vi "createSegment.vi"(4 "log":string, 5 "time":string, 6 "Parameter":string[][](array[string]), 7 "Comment":string, 8 "error in (no error)":errorcluster, 9 "SegName":string, 10 "test ref":refnum<k20>, 11 "DOM document":refnum<k20>) -> (0 "error out":errorcluster, 1 "seg ref":refnum<k20>, 2 "dup test ref":refnum<k20>, 3 "dup DOM document":refnum<k20>)   [LabVIEW 2013, in "XML.lvlib"]
uses:
  lib/XML.lvlib
  <vilib>/xml/Close Reference(Node).vi
  <resource>/objmgr/DOMUserDefRef.rc
  <vilib>/xml/NI_XML.lvlib
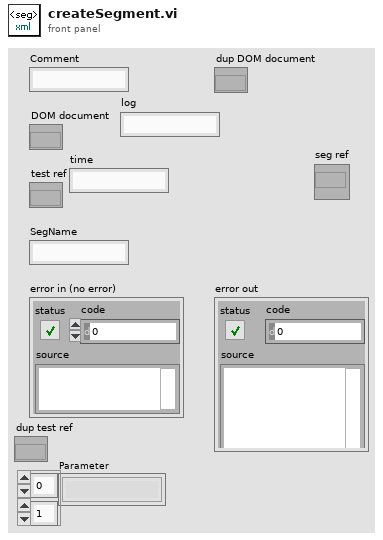
[diagram p1: front panel]
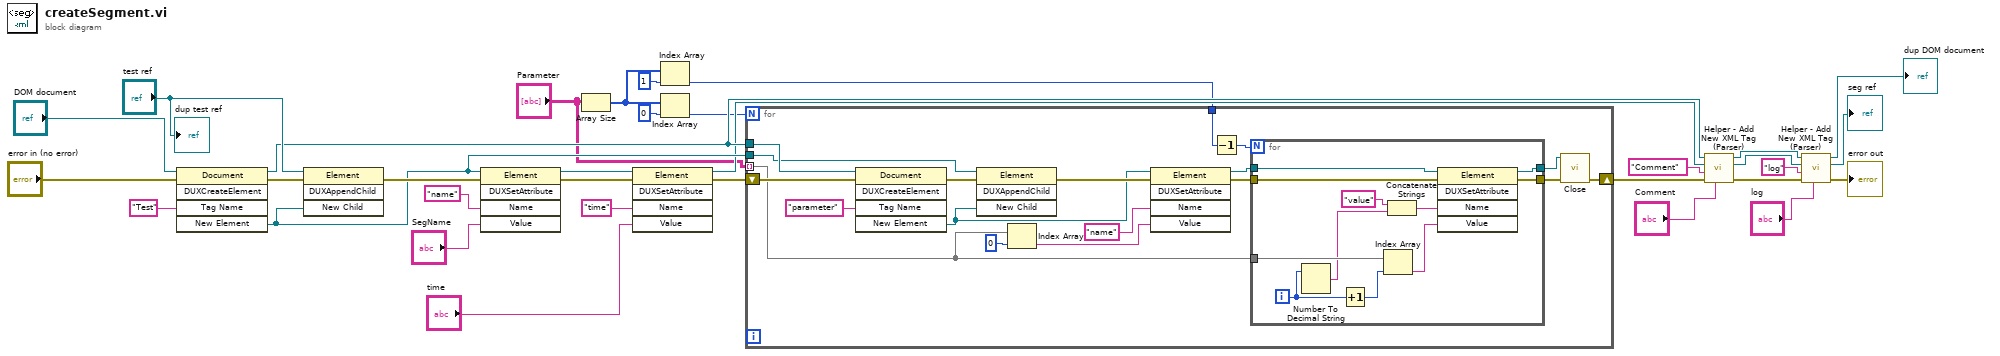
[diagram p0: block diagram]
diagram:
  n1 = invoke class="Document" method="DUXCreateElement"(reference="DOM document", error in="error in (no error)", "Tag Name"="Test") -> (reference out=w11:refnum<k20>, error out=w31:errorcluster, "New Element"=w8:refnum<k20>)  [unwired: 2 in, 2 out]
  n2 = invoke class="Element" method="DUXAppendChild"(reference="test ref", error in=w31, "New Child"=w8) -> (error out=w27:errorcluster)  [unwired: 1 in, 3 out]
  n3 = invoke class="Element" method="DUXSetAttribute"(reference=w8, error in=w27, "Name"="name" ("Tag Name"), "Value"="SegName") -> (reference out=w22:refnum<k20>, error out=w23:errorcluster)  [unwired: 1 in, 3 out]
  n4 = Array Size(array="Parameter") -> (size(s)=w2:i32[])
  n5 = invoke class="Element" method="DUXSetAttribute"(reference=w22, error in=w23, "Name"="time" ("Tag Name"), "Value"="time") -> (reference out=w7:refnum<k20>, error out=w10:errorcluster)  [unwired: 1 in, 3 out]
  n6 = Index Array(array=w2, index=1 ("Index")) -> (element=w1:i32)
  n7 = Index Array(array=w2, index=0 ("Index")) -> (element=w4:i32)
  n8 = for {
    N: w4 -> [_]
    tunnel: "Parameter" -> [w36] mode=indexing
    tunnel: w11 -> [w45]
    shift-right: [w37] -> w9
    shift-left: w10 -> [w44]
    tunnel: w8 -> [w43]
    tunnel: w1 -> [w34]
    n9 = invoke class="Document" method="DUXCreateElement"(reference=w45, error in=w44, "Tag Name"="parameter") -> (error out=w50:errorcluster, "New Element"=w42:refnum<k20>)  [unwired: 2 in, 3 out]
    n10 = invoke class="Element" method="DUXAppendChild"(reference=w43, error in=w50, "New Child"=w42) -> (error out=w46:errorcluster)  [unwired: 1 in, 3 out]
    n11 = Index Array(array=w36, index=0 ("Index")) -> (element=w40:string)
    n12 = invoke class="Element" method="DUXSetAttribute"(reference=w42, error in=w46, "Name"="name" ("Tag Name"), "Value"=w40) -> (reference out=w49:refnum<k20>, error out=w48:errorcluster)  [unwired: 1 in, 3 out]
    n13 = Decrement(x=w34) -> (x-1=w35:i32)
    n14 = for {
      N: w35 -> [_]
      tunnel: w49 -> [w62]
      tunnel: w48 -> [w61]
      tunnel: [w59] -> w39
      tunnel: [w58] -> w38
      tunnel: w36 -> [w57]
      i -> [w53]
      n15 = Number To Decimal String(number=w53) -> (decimal integer string=w54:string)  [unwired: 1 in]
      n16 = Increment(x=w53) -> (x+1=w55:i32)
      n17 = Index Array(array=w57, index=w55) -> (element=w60:string)
      n18 = Concatenate Strings("value" ("Tag Name"), w54) -> (w52:string)
      n19 = invoke class="Element" method="DUXSetAttribute"(reference=w62, error in=w61, "Name"=w52, "Value"=w60) -> (reference out=w58:refnum<k20>, error out=w59:errorcluster)  [unwired: 1 in, 3 out]
    }
    n20 = call-poly <vilib>:"Close.vi"("error in (no error)"=w39, "node"=w38) -> ("error out"=w37:errorcluster)  [unwired: 7 out]
  }
  n21 = call "Helper - Add New XML Tag (Parser).vi"("Tag Data"="Comment", "error in (no error)"=w9, "Tag Name"="Comment", "Owning Element"=w7, "DOM document"=w11) -> ("error out"=w16:errorcluster, "dup Owning Element"=w18:refnum<k20>, "dup DOM document"=w19:refnum<k20>)  [unwired: 4 in]
  n22 = call "Helper - Add New XML Tag (Parser).vi"("Tag Data"="log", "error in (no error)"=w16, "Tag Name"="log", "Owning Element"=w18, "DOM document"=w19) -> ("error out"=→"error out":errorcluster, "dup Owning Element"=→"seg ref":refnum<k20>, "dup DOM document"=→"dup DOM document":refnum<k20>)  [unwired: 4 in]
  "dup test ref" <- "test ref"
